vi "Configure ET Delay Step.vi"(8 "error in (no error)":errorcluster, 11 "Servo MSMT in":refnum<class "Servo MSMT.lvclass">) -> (0 "error out":errorcluster, 3 "Servo MSMT out":refnum<class "Servo MSMT.lvclass">)   [LabVIEW 2018, in "Servo MSMT.lvlib" / "Servo MSMT.lvclass"]
uses:
  Servo MSMT.lvclass
  C:/Sequence Automation/Plugins/Measurement Interface.lvlibp/Measurement Interface.lvclass
  Plugins/Measurement Interface.lvlibp/Private Methods/Measurement Name/Read Measurement Name.vi
  Plugins/TestStand API Tools (TSAT).lvlibp/Step Actions/TSAT Step Actions.lvlib
  Plugins/Measurement Interface.lvlibp/Measurement Interface.lvclass
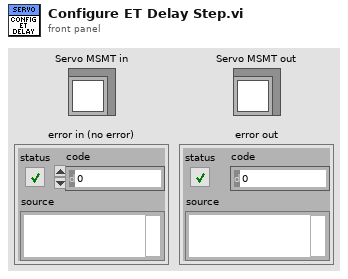
[diagram p1: front panel]
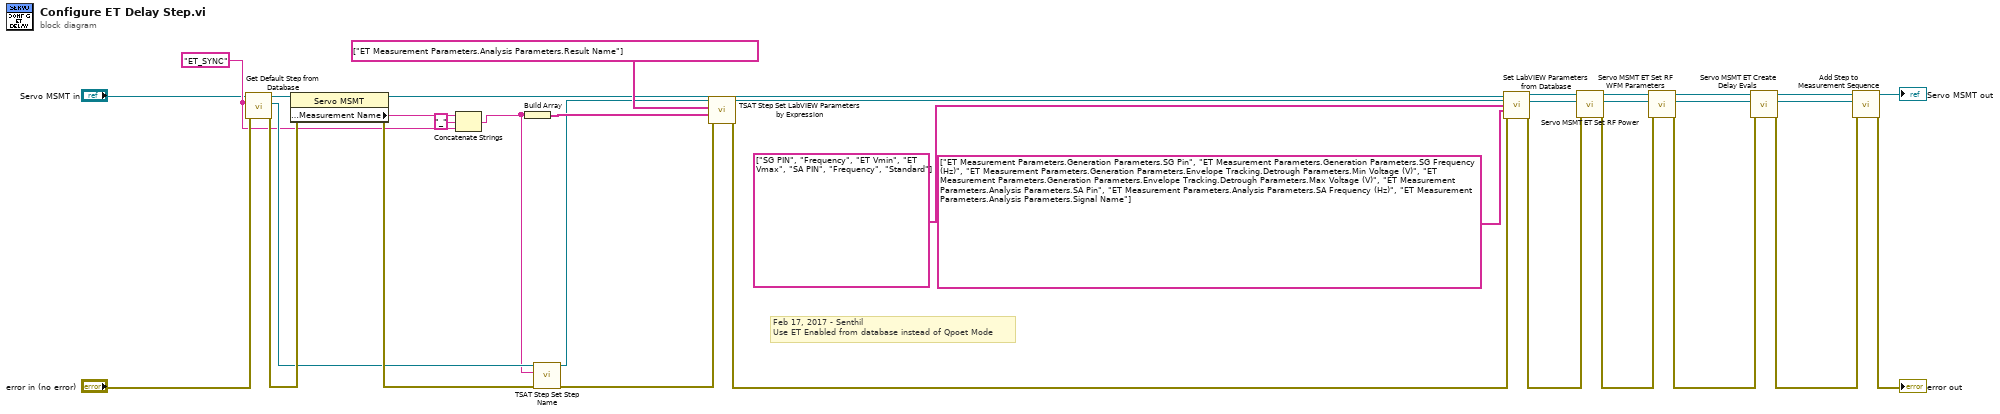
[diagram p0: block diagram]
diagram:
  w9 = "ET_SYNC" ("Standard")
  # "Feb 17, 2017 - Senthil\nUse ET Enabled from database instead of Qpoet Mode"
  n1 = call "Get Default Step from Database.vi"("error in (no error)"="error in (no error)", "Default Step"=w9, "Measurement Interface in"="Servo MSMT in") -> ("error out"=w17:errorcluster, "Cloned Step"=w11:refnum<k7>, "Measurement Interface out"=w21:refnum<class "Servo MSMT.lvclass">)  [unwired: 6 in]
  n2 = property class="Servo MSMT"(reference=w21, error in=w17) -> (reference out=w20:refnum<class "Servo MSMT.lvclass">, error out=w16:errorcluster, "Public Methods:Measurement Name"=w19:string)
  n3 = Concatenate Strings(w19, "_" ("string"), w9) -> (w8:string)
  n4 = Build Array(w8) -> (w33:string[])
  n5 = call "TSAT Step Set Step Name.vi"("Error In"=w16, "Name"=w8, "Step In"=w11) -> ("Error Out"=w12:errorcluster, "Step Out"=w10:refnum<k7>)  [unwired: 7 in]
  n6 = call "TSAT Step Set LabVIEW Parameters by Expression.vi"("Error In"=w12, "Value Expressions"=w33, "Parameters to Set"=string[] ["ET Measurement Parameters.Analysis Parameters.Result Name"], "Step In"=w10) -> ("Error Out"=w31:errorcluster, "Step Out"=w30:refnum<k7>)  [unwired: 6 in]
  n7 = call "Set LabVIEW Parameters from Database.vi"("Measurement Interface in"=w20, "Step In"=w30, "Dictionary Keys"=string[] ["SG PIN", "Frequency", "ET Vmin", "ET Vmax", "SA PIN", "Frequency", "Standard"] ("Database Keys"), "LabVIEW Parameter Mapping"=string[] ["ET Measurement Parameters.Generation Parameters.SG Pin", "ET Measurement Parameters.Generation Parameters.SG Frequency (Hz)", "ET Measurement Parameters.Generation Parameters.Envelope Tracking.Detrough Parameters.Min Voltage (V)", "ET Measurement Parameters.Generation Parameters.Envelope Tracking.Detrough Parameters.Max Voltage (V)", "ET Measurement Parameters.Analysis Parameters.SA Pin", "ET Measurement Parameters.Analysis Parameters.SA Frequency (Hz)", "ET Measurement Parameters.Analysis Parameters.Signal Name"] ("Database Keys"), "error in (no error)"=w31) -> ("Measurement Interface out"=w15:refnum<class "Servo MSMT.lvclass">, "Step Out"=w13:refnum<k7>, "error out"=w14:errorcluster)  [unwired: 8 in]
  n8 = call-dynamic "Servo MSMT ET Set RF Power.vi"("error in (no error)"=w14, "Step In"=w13, "Servo MSMT in"=w15) -> ("error out"=w22:errorcluster, "Step Out"=w23:refnum<k7>, "Servo MSMT out"=w24:refnum<class "Servo MSMT.lvclass">)  [unwired: 6 in]
  n9 = call "Servo MSMT ET Set RF WFM Parameters.vi"("error in (no error)"=w22, "Step In"=w23, "Servo MSMT in"=w24) -> ("error out"=w27:errorcluster, "Step Out"=w3:refnum<k7>, "Servo MSMT out"=w5:refnum<class "Servo MSMT.lvclass">)  [unwired: 6 in]
  n10 = call "Servo MSMT ET Create Delay Evals.vi"("error in (no error)"=w27, "Step In"=w3, "Servo MSMT in"=w5) -> ("error out"=w6:errorcluster, "Step Out"=w2:refnum<k7>, "Servo MSMT out"=w4:refnum<class "Servo MSMT.lvclass">)  [unwired: 6 in]
  n11 = call "Add Step to Measurement Sequence.vi"("error in (no error)"=w6, "Step to Add"=w2, "Measurement Interface in"=w4) -> ("error out"=→"error out":errorcluster, "Measurement Interface out"=→"Servo MSMT out":refnum<class "Servo MSMT.lvclass">)  [unwired: 7 in]
